vi "Update Plugins Data.vi"(8 "error in (no error)":errorcluster, 10 "Plugins":refnum<class "Plugin.lvclass">[](array[class]), 11 "Logging Thread in":refnum<class "Logging Thread.lvclass">) -> (0 "error out":errorcluster, 3 "Logging Thread out":refnum<class "Logging Thread.lvclass">)   [LabVIEW 2017, in "DSF Core.lvlib" / "Logging Thread.lvclass"]
uses:
  Logging Thread.lvclass
  Plugin/Plugin.lvclass
  Plugin Data.ctl
  Logging Thread.lvclass/Logging Thread.ctl
  Pool/Plugin Interface/Plugin Interface Pool.lvclass
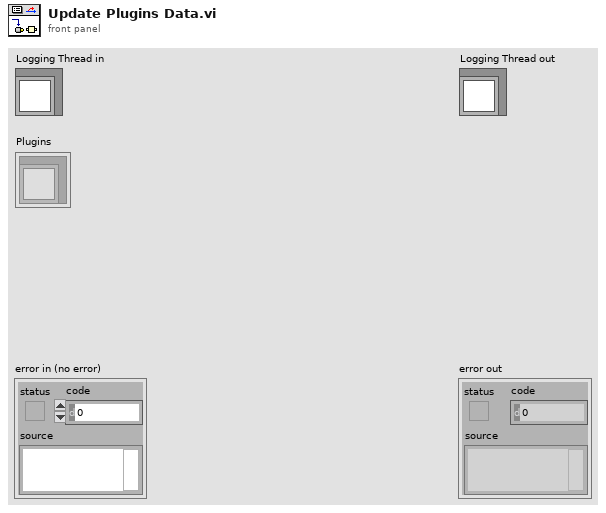
[diagram p1: front panel]
types:
  T1 = typedef "DSF Core.lvlib/Logging Thread.lvclass/Plugin Data.ctl" = cluster{"thread names":string[]}
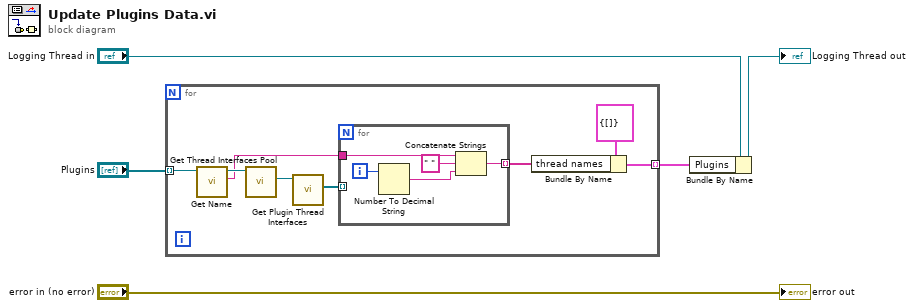
[diagram p0: block diagram]
diagram:
  n1 = for {
    tunnel: "Plugins" -> [w12] mode=indexing
    tunnel: [w9] -> w3 mode=indexing
    n2 = call "Get Name.vi"("Plugin in"=w12) -> ("name"=w7:string, "Plugin out"=w11:refnum<class "Plugin.lvclass">)  [unwired: 9 in]
    n3 = call "Get Thread Interfaces Pool.vi"("Plugin in"=w11) -> ("Plugin Interfaces Pool"=w10:refnum<class "Plugin Interface Pool.lvclass">)  [unwired: 9 in, 1 out]
    n4 = call "Get Plugin Thread Interfaces.vi"("Plugin Interface Pool in"=w10) -> ("Plugin Thread Interfaces"=w8:refnum<class "Plugin Interface.lvclass">[])  [unwired: 9 in, 1 out]
    n5 = for {
      tunnel: w8 -> [_] mode=indexing
      tunnel: w7 -> [w17]
      tunnel: [w16] -> w6 mode=indexing
      i -> [w18]
      n6 = Number To Decimal String(number=w18) -> (decimal integer string=w15:string)  [unwired: 1 in]
      n7 = Concatenate Strings(w17, " " ("string"), w15) -> (w16:string)
    }
    n8 = Bundle By Name(cluster=T1 {"thread names"=[]} ("plugin data"), "thread names"=w6) -> (w9:T1)
  }
  n9 = Bundle By Name(cluster="Logging Thread in", "Plugins"=w3) -> (→"Logging Thread out":refnum<class "Logging Thread.lvclass">)
  "error out" <- "error in (no error)"
